vi "PCA ReadMeanSize.vi"(8 "error in (no error)":errorcluster, 11 "PCA in":refnum<class "PCA.lvclass">) -> (0 "error out":errorcluster, 1 "cols":i32, 2 "rows":i32, 3 "PCA out":refnum<class "PCA.lvclass">)   [LabVIEW 2020, in "OpenLvVision_OpenCv.lvlib" / "PCA.lvclass"]
doc: "Retruns the size of mean matrix."
uses:
  PCA.lvclass
  C:/Users/lukas/Downloads/OpenLvVision_OpenCv/SourceCode/LabView/OpenLvVision_OpenCv/_LvHelpers/EdvrObject/EdvrObject.lvclass
  _LvHelpers/EdvrObject/EdvrObject.lvclass/EdvrObject.ctl
  OpenLvVision_OpenCv.lvlib
  _LvHelpers/EdvrObject/EdvrObject.lvclass
  Dlls/OlvOpenCvWrapper.dll
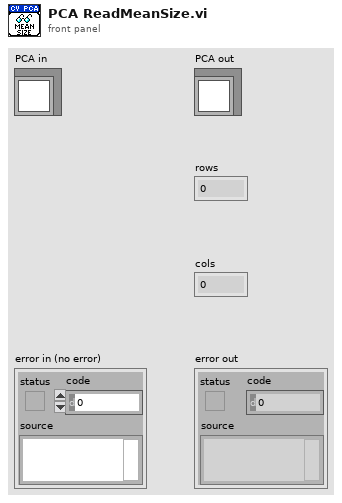
[diagram p1: front panel]
types:
  T1 = typedef "OpenLvVision_OpenCv.lvlib/EdvrObject.lvclass/Edvr.ctl" = refnum<data-value>
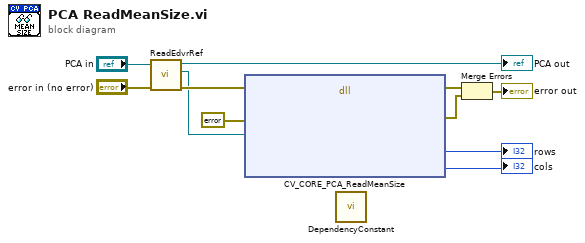
[diagram p0: block diagram]
diagram:
  n1 = call "ReadEdvrRef.vi"("error in (no error)"="error in (no error)", "EdvrObject in"="PCA in") -> ("error out"=w7:errorcluster, "Edvr"=w3:T1, "EdvrObject out"=→"PCA out":refnum<class "PCA.lvclass">)  [unwired: 7 in]
  n2 = dll-call lib="C:/Users/lukas/Downloads/OpenLvVision_OpenCv/SourceCode/LabView/OpenLvVision_OpenCv/Dlls/OlvOpenCvWrapper.dll" fn="CV_CORE_PCA_ReadMeanSize"(error in=w7, "Error"=errorcluster {"status"=FALSE, "code"=0, "source"=""} ("error out"), "edvrRef"=w3) -> (error out=w8:errorcluster, "Error"=w6:errorcluster, "rows"=→"rows":i32, "cols"=→"cols":i32)  [unwired: 6 in, 1 out]
  n3 = call "DependencyConstant.vi"() -> ()  [unwired: 12 in]
  n4 = Merge Errors(w8, w6) -> (→"error out":errorcluster)
